vi "Enstack Queue.vi"(8 "error in (no error)":errorcluster, 10 "State":string, 11 "queue ref":refnum<queue>) -> (0 "error out":errorcluster, 3 "queue out":refnum<queue>)   [LabVIEW 2022 SP3]
doc: "Use this template to build a VI to use as a subVI."
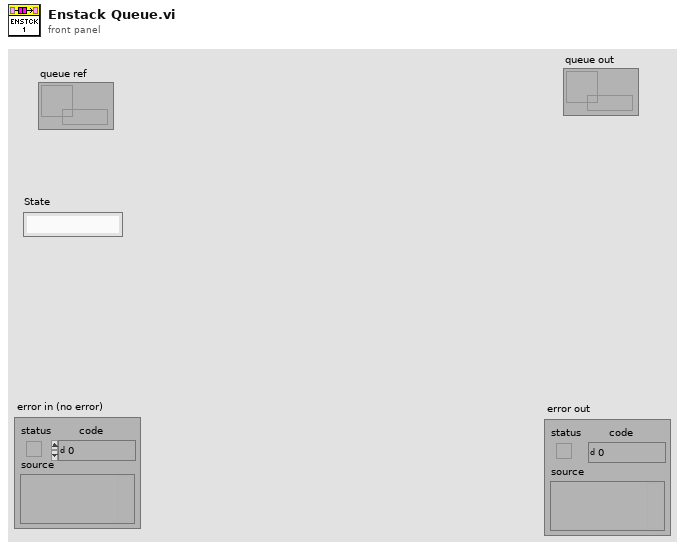
[diagram p1: front panel]
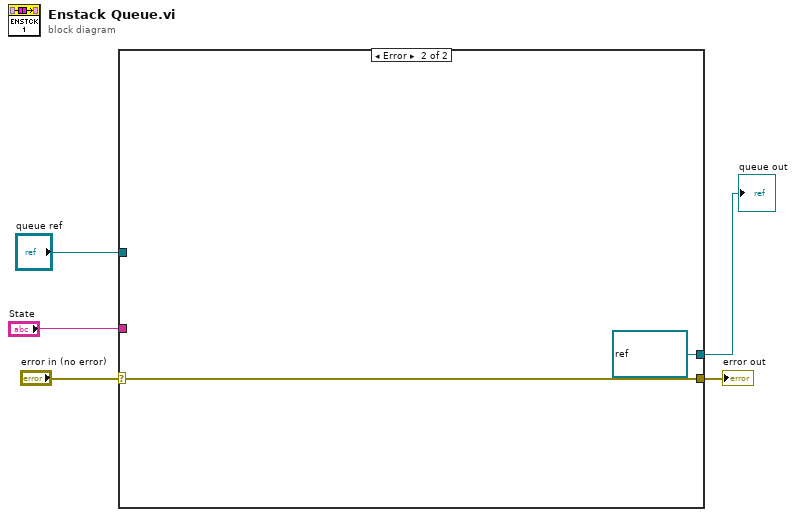
[diagram p0: block diagram]
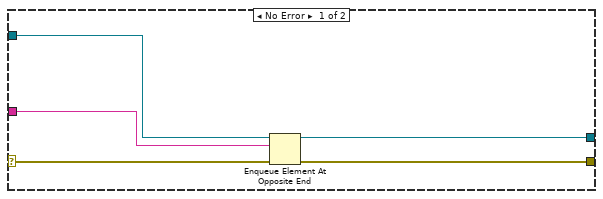
[diagram p2: hidden frame]
diagram:
  n1 = case shown="Error" "error in (no error)" {
    selector: "error in (no error)" -> [w10 w12]
    tunnel: [w9 w12] -> w4
    tunnel: "queue ref" -> [w8 _]
    tunnel: "State" -> [w7 _]
    tunnel: [w6 refnum<queue> refnum ("queue ref")] -> w1
    frame No Error {
      n2 = Enqueue Element At Opposite End(queue=w8, element=w7, error in (no error)=w10) -> (queue out=w6:refnum<queue>, error out=w9:errorcluster)  [unwired: 1 in, 1 out]
    }
    frame Error {
    }
  }
  "error out" <- w4
  "queue out" <- w1
